vi "AddMouseState.vi"(8 "error in (no error)":errorcluster, 10 "New Mouse State":T1, 11 "Input in":refnum<class "Input.lvclass">) -> (0 "error out":errorcluster, 3 "Input out":refnum<class "Input.lvclass">)   [LabVIEW 2015]
uses:
  Input.lvclass
  Mouse State.ctl
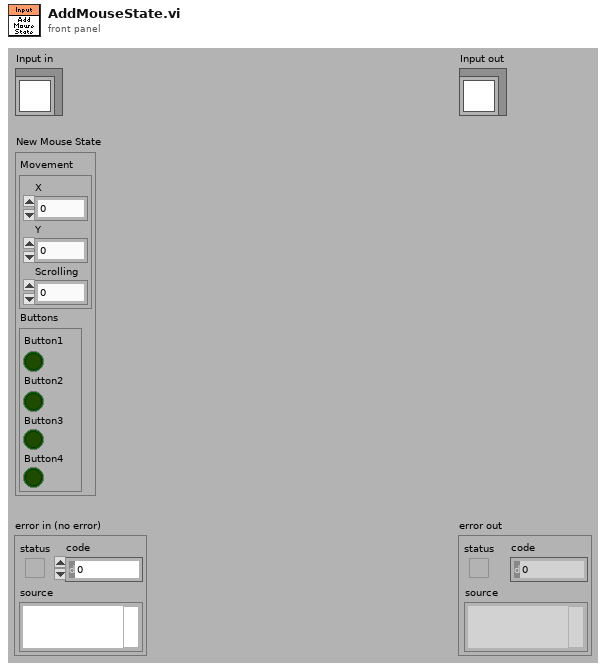
[diagram p1: front panel]
types:
  T1 = typedef "Input.lvclass/Mouse State.ctl" = cluster{"Movement":cluster{"X":i32, "Y":i32, "Scrolling":i32}, "Buttons":cluster{"Button1":bool, "Button2":bool, "Button3":bool, "Button4":bool}}
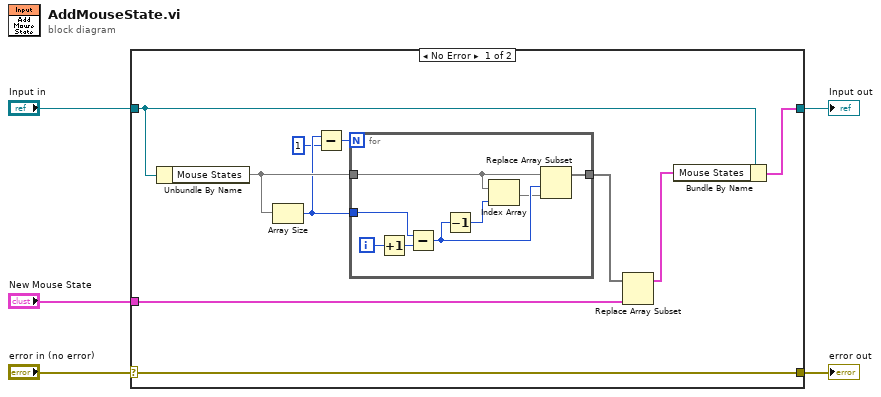
[diagram p0: block diagram]
diagram:
  n1 = case shown="No Error" "error in (no error)" {
    selector: "error in (no error)" -> [w15 w25]
    tunnel: [w15 w25] -> w4
    tunnel: [w7 w24] -> w2
    tunnel: "Input in" -> [w8 w24]
    tunnel: "New Mouse State" -> [w9 _]
    frame No Error {
      n2 = Unbundle By Name(w8) -> ("Mouse States"=w14)
      n3 = Array Size(array=w14) -> (size(s)=w13:i32)
      n4 = Subtract(x=w13, y=1 ("x")) -> (x-y=w12:i32)
      n5 = for {
        N: w12 -> [_]
        tunnel: w14 -> [w21]
        tunnel: w13 -> [w17]
        tunnel: [w16] -> w10
        i -> [w23]
        n6 = Increment(x=w23) -> (x+1=w22:i32)
        n7 = Subtract(x=w17, y=w22) -> (x-y=w20:i32)
        n8 = Decrement(x=w20) -> (x-1=w19:i32)
        n9 = Index Array(array=w21, index=w19) -> (element=w18)
        n10 = Replace Array Subset(array=w21, new element=w18, index=w20) -> (w16:void[])
      }
      n11 = Replace Array Subset(array=w10, new element=w9) -> (w6:T1[])  [unwired: 1 in]
      n12 = Bundle By Name(cluster=w8, "Mouse States"=w6) -> (w7:cluster{})
    }
    frame Error {
    }
  }
  "error out" <- w4
  "Input out" <- w2
